vi "STC_Starrag_main_V3.vi"() -> ()   [LabVIEW 2017]
uses:
  controls/FPGA State.ctl
  controls/UI Data2.ctl
  controls/Chatter data.ctl
  Globals/Global - All UI Loop Stop.vi
  Globals/Global - UI Stream and Variable Connections.vi
  Globals/Global - Configuration Options.vi
  UI Error Handlers/support/User Event - Stop/User Event - Stop.lvlib
  UI Error Handlers/support/Message Queue/Message Queue.lvlib
panel:
  out "Raw Waveform":waveform(dbl)[](graph)
  in  "Settings Tab":T1(tab)=enum."Data Monitoring"
  in  "OK Button":bool
  in  "Tool Data File":path=path "K:/Core Research/Project Folders/AI Projects/AI3190 Digital Shop Floor Rollout/5 Software Files/Catapult/tool_path.txt"
  in  "Run Control":bool
  in  "Stop Control":bool
  in  "Max Acceleration Threshold (g)":sgl=0.03
  in  "In-cut Power Threshold":dbl=1.0
  in  "Controller Address":string="143.167.158.195"
  in  "Connect to Controller":bool
  out "Connected?":bool
  out "System Status":string
  in  "Save?":bool
  in  "Switch to Safe State":bool
  out "Current FPGA State":T2
  out "Tool Data":string="\n"
  in  "ODBC data source name":string="amrc_monitoring"
  in  "MT Connect Agent":string="http://amrcmtconnect.shef.ac.uk:5000/"
  in  "milliseconds to wait":u32=100
  in  "Machine":string="STC1250"
  out "Loop execution":u32
  out "output cluster":cluster{"G1 ":bool}
  out "tag acc":string
  out "tag spike":string
  out "Chatter?":bool
  out "Feed":dbl
  out "ACC  (grms)":T3(graph)
  out "Block of code being executed":string
  out "Program Name":string
  out "RPM":dbl
  out "STC Starrag":bool
  out "Force (grms)":T4(graph)
  out "Tool id":string
  out "Spindle Load":dbl[](graph)
  out "CPU Usage (%)":dbl[][](graph)
  out "Free Physical Memory or Largest Contiguous Memory (bytes)":dbl(graph)
  out "DMA FIFO Overflow?":bool
  in  "Exit":bool
  # "Acceleration Waveform for 0.5s"
  # "Connection Settings"
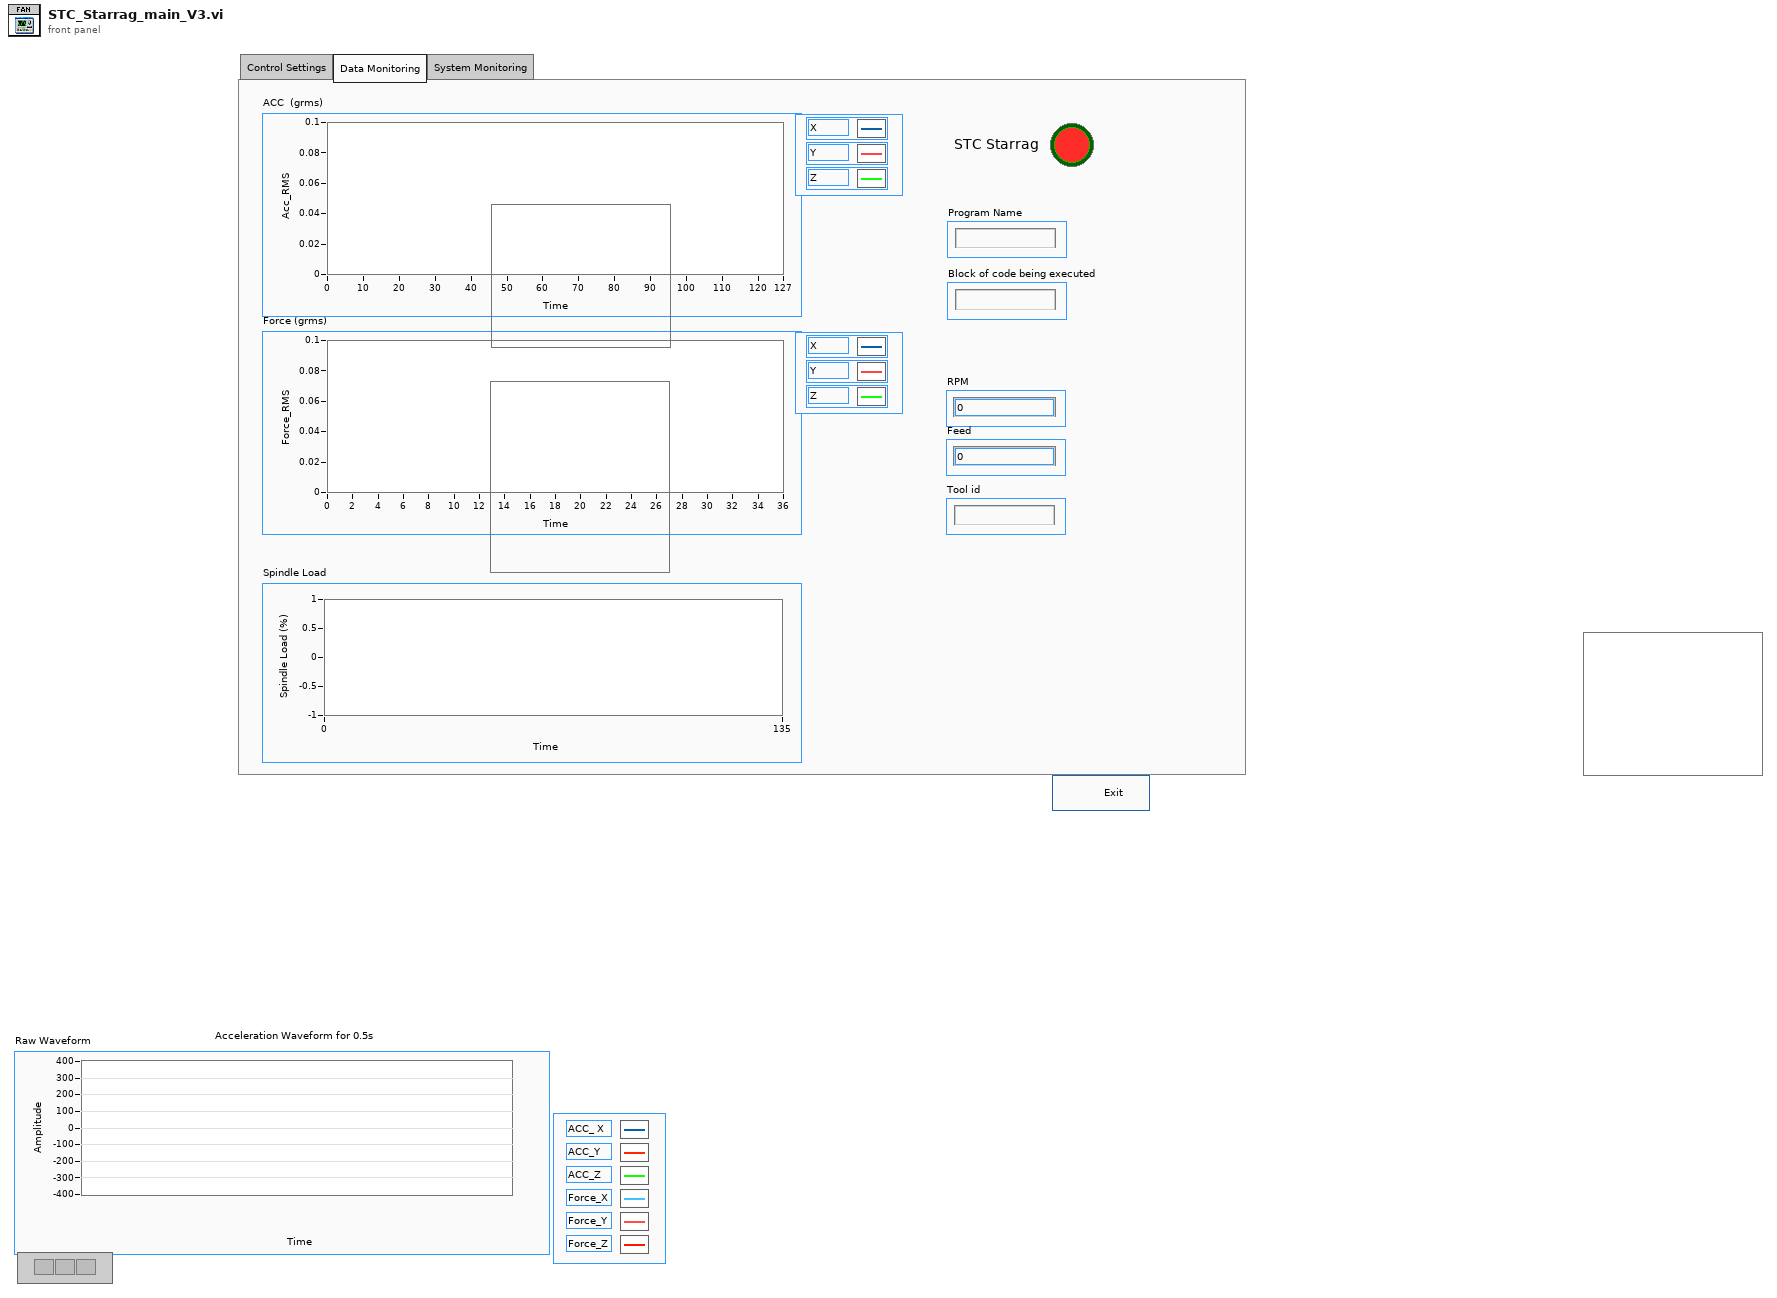
[diagram p1: front panel]
types:
  T1 = enum32{"Control Settings", "Data Monitoring", "System Monitoring"}
  T2 = typedef "FPGA State.ctl" = enum16{"Safe State", "Control (PID)"}
  T3 = cluster{"Array of Double[0]":dbl, "Array of Double[1]":dbl, "Array of Double[2]":dbl}
  T4 = cluster{"[0]":dbl, "[1]":dbl, "[2]":dbl, "[3]":dbl, "[4]":dbl, "[5]":dbl, "[6]":dbl, "[7]":dbl}
  T5 = typedef "UI Data2.ctl" = cluster{"Switch to Safe State Ref":refnum<vi>, "Run Control Ref":refnum<vi>, "Stop Control Ref":refnum<vi>, "Update Control Configurations Ref":refnum<vi>, "Chatter Data Ref":refnum<vi>, "Max Acceleration Threshold Ref":refnum<vi>}
  T6 = typedef "Message Queue.lvlib/All Message Queues.ctl" = cluster{"UI":refnum<queue>}
  T7 = enum8{"Enabled", "Disabled", "Disabled and Grayed Out"}
  T8 = cluster{"Message":string, "Message Data":variant}
  T9 = typedef "Chatter data.ctl" = cluster{"Tool data":cluster{"Number of teeth":sgl}, "Cutting data":cluster{"rpm":sgl}, "Limits":cluster{"Magnitude threshold":sgl, "Tolerance":sgl}, "G1 status":cluster{"G1 ":bool}}
  T10 = cluster{"FPGA State":T2, "Max Acceleration Threshold":sgl, "Chatter Data":T9}
  T11 = cluster{"seconds since 1Jan1904":timestamp, "number":dbl[][], "Machine Data":cluster{"Zload":string, "Yload":string, "Xload":string, "path_position":string, "Fovr":string, "SspeedOvr":string, "Program Name":string, "Program status":string, "Block of code being executed":string, "Line of code":string, "Machine availability":string, "Emergency status":string, "Controller mode":string, "Tool_id":string}}
  T12 = cluster{"seconds since 1Jan1904":timestamp, "number":dbl[][], "Machine Data":cluster{"Zload":string, "Yload":string, "Xload":string, "path_position":string, "Fovr":string, "SspeedOvr":string, "Program Name":string, "Program status":string, "Block of code being executed":string, "Line of code":string, "Machine availability":string, "Emergency status":string, "Controller mode":string, "Tool id":string}}
  T13 = cluster{"Actual PID Loop Period":refnum<k21>, "DMA FIFO Overflow?":refnum<k21>, "CPU Usage":refnum<k21>, "Free or Contiguous Memory":refnum<k21>, "Current FPGA State":refnum<k21>, "Acceleration (grms)":refnum<k21>, "Acceleration Waveform":refnum<k21>, "Chatter":refnum<k21>, "tag acc":refnum<k21>, "tag video":refnum<k21>, "Image Waveform":refnum<k21>}
  T14 = cluster{"Zload":string, "Yload":string, "Xload":string, "path_position":string, "Fovr":string, "SspeedOvr":string, "Program Name":string, "Program status":string, "Block of code being executed":string, "Line of code":string, "Machine availability":string, "Emergency status":string, "Controller mode":string, "Tool_id":string}
  T15 = cluster{"Zload":string, "Yload":string, "Xload":string, "path_position":string, "Fovr":string, "SspeedOvr":string, "Program Name":string, "Program status":string, "Block of code being executed":string, "Line of code":string, "Machine availability":string, "Emergency status":string, "Controller mode":string, "Tool id":string}
  T16 = cluster{"Magnitude threshold":sgl, "Tolerance":sgl}
  T17 = typedef "FPGA state.ctl" = enum16{"Safe State", "Control (PID)"}
  T18 = typedef "CPU Loads.ctl" = cluster{"Total (%)":dbl, "Time Critical (%)":dbl, "Timed Structures (%)":dbl, "High (%)":dbl, "Above Normal (%)":dbl, "Normal (%)":dbl, "Background (%)":dbl, "Idle (%)":dbl, "ISR (%)":dbl}[]
  T19 = cluster{"seconds since 1Jan1904":timestamp, "appended array":dbl[][], "Machine Data":cluster{"Zload":string, "Yload":string, "Xload":string, "path_position":string, "Fovr":string, "SspeedOvr":string, "Program Name":string, "Program status":string, "Block of code being executed":string, "Line of code":string, "Machine availability":string, "Emergency status":string, "Controller mode":string, "Tool_id":string}}
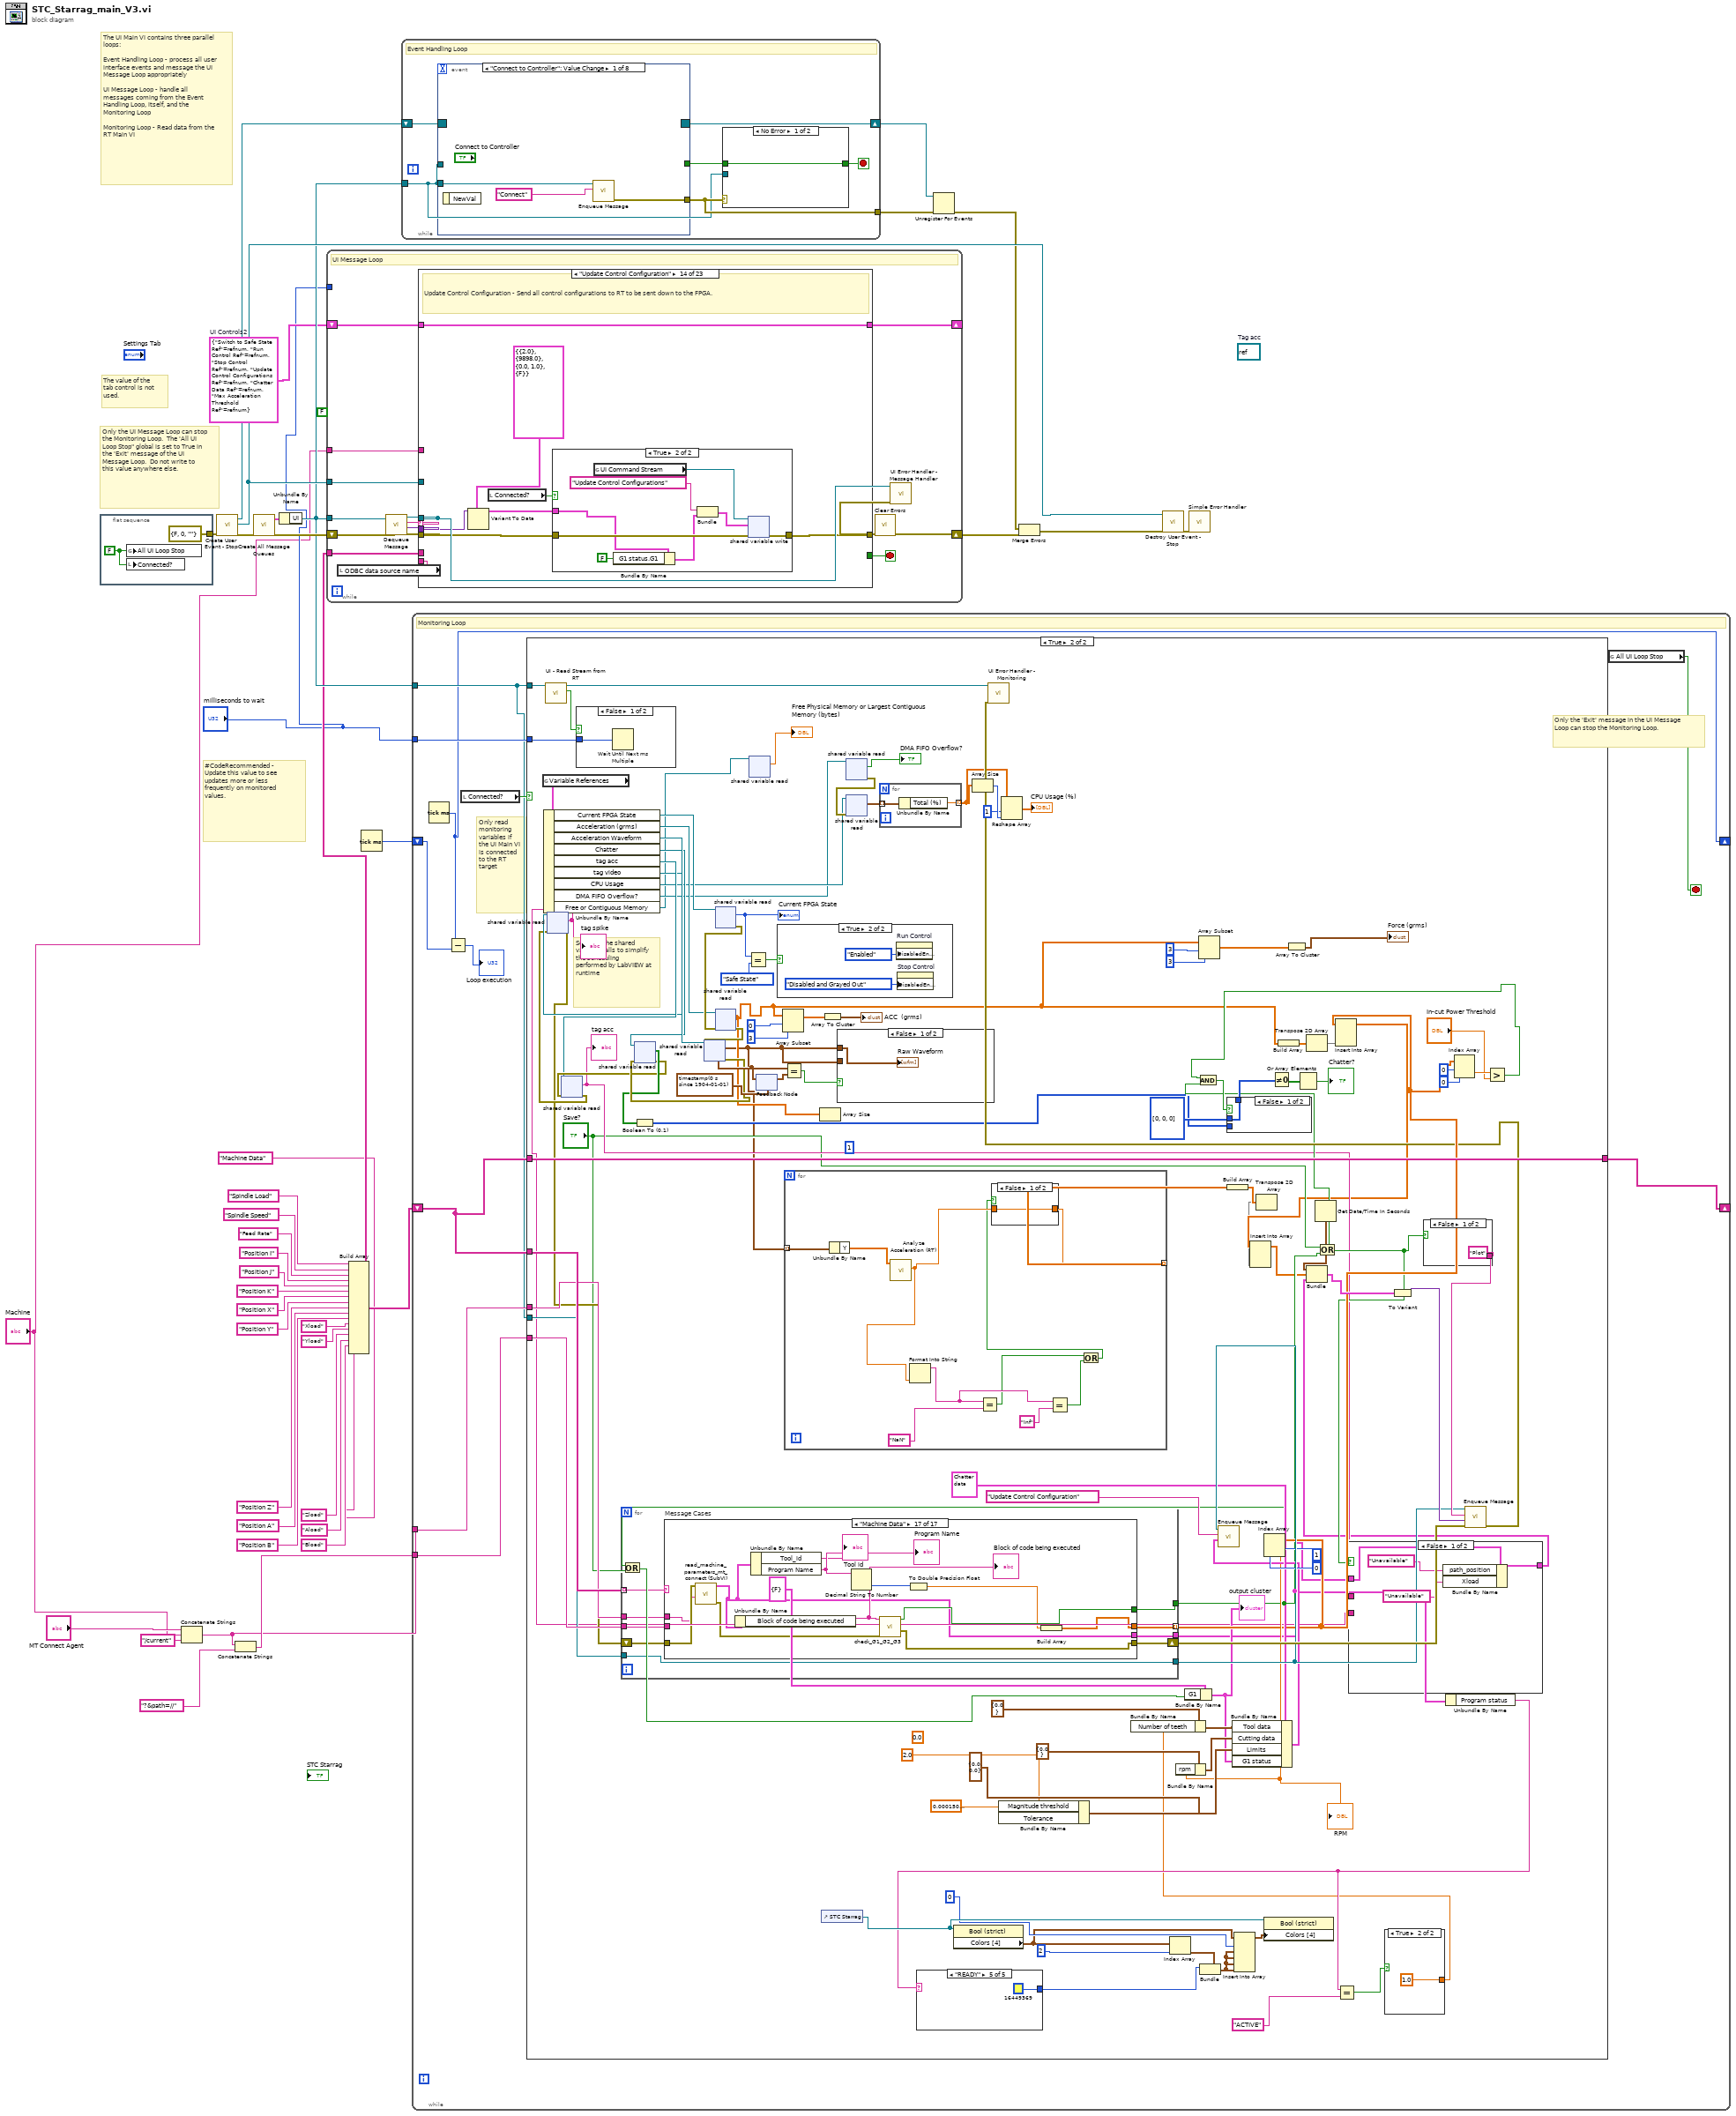
[diagram p0: block diagram]
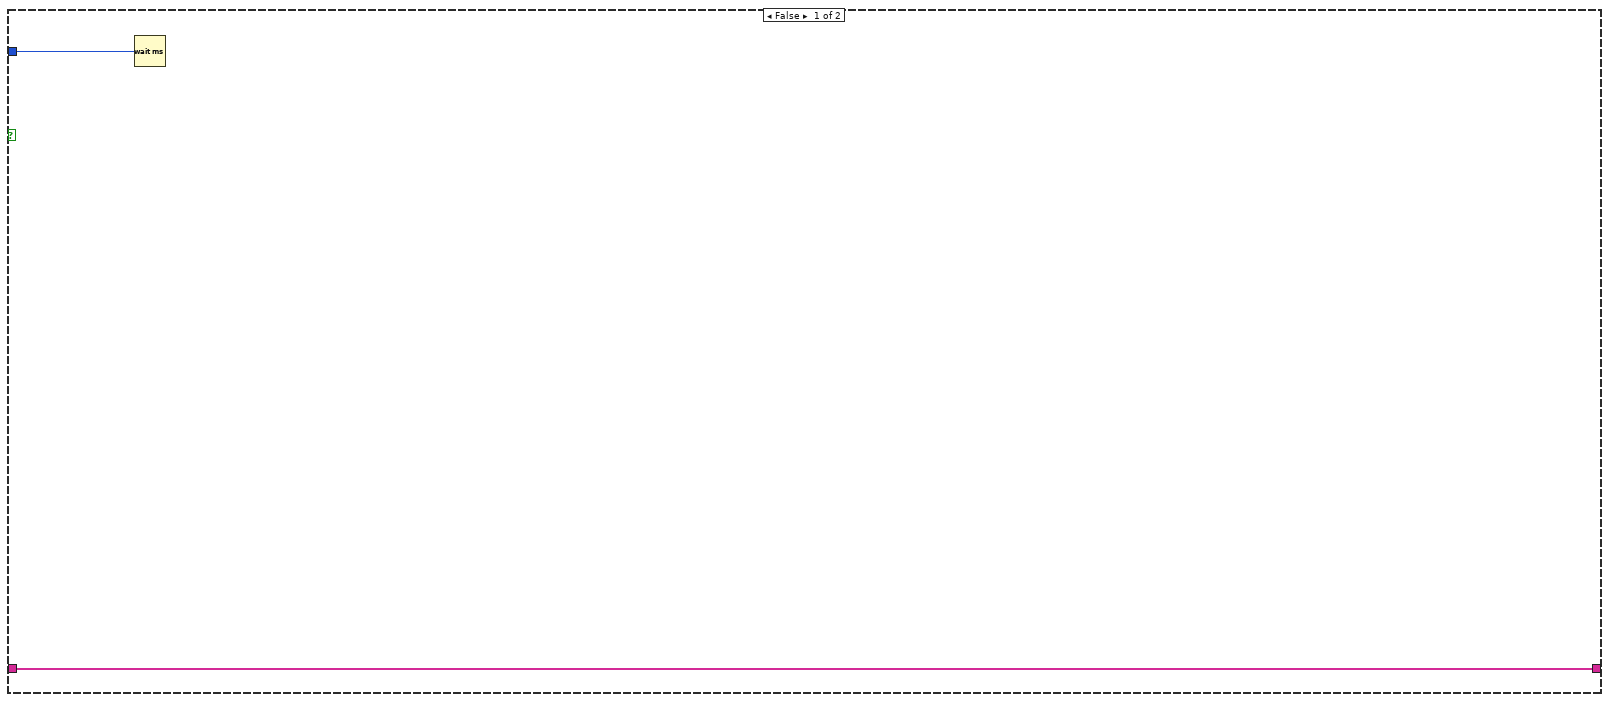
[diagram p2: hidden frame]
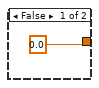
[diagram p3: hidden frame]
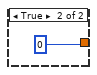
[diagram p4: hidden frame]
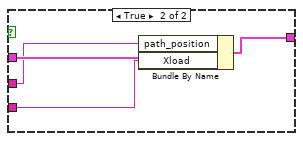
[diagram p5: hidden frame]
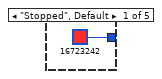
[diagram p6: hidden frame]
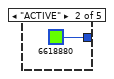
[diagram p7: hidden frame]
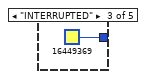
[diagram p8: hidden frame]
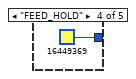
[diagram p9: hidden frame]
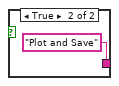
[diagram p11: hidden frame]
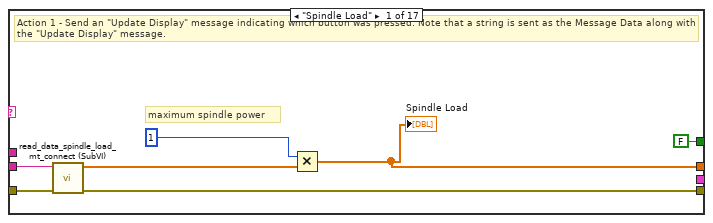
[diagram p12: hidden frame]
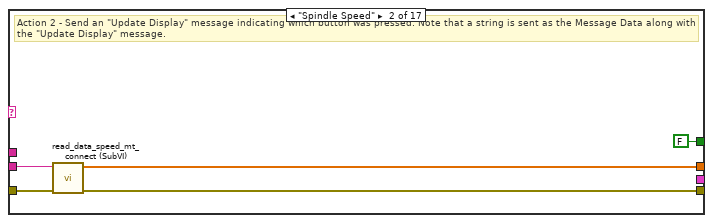
[diagram p13: hidden frame]
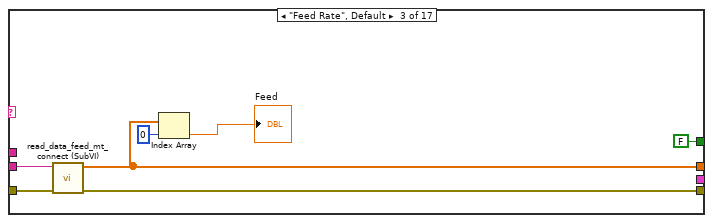
[diagram p14: hidden frame]
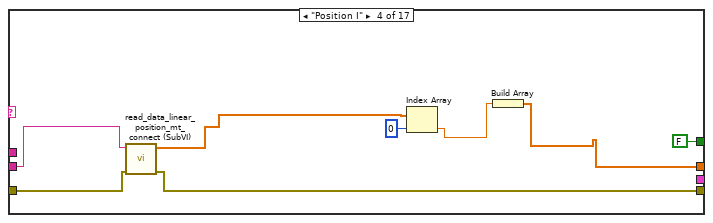
[diagram p15: hidden frame]
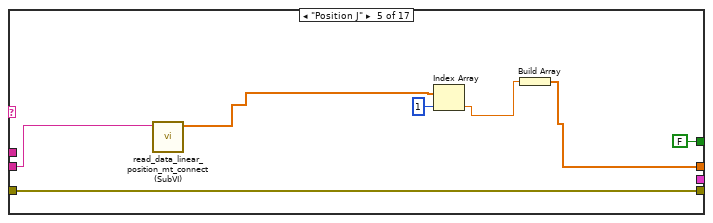
[diagram p16: hidden frame]
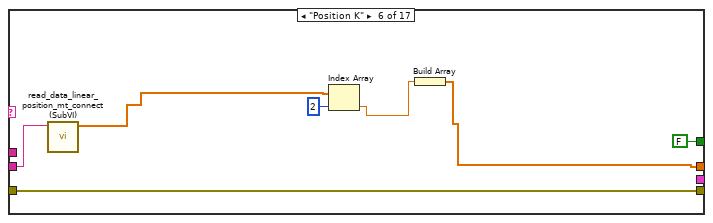
[diagram p17: hidden frame]
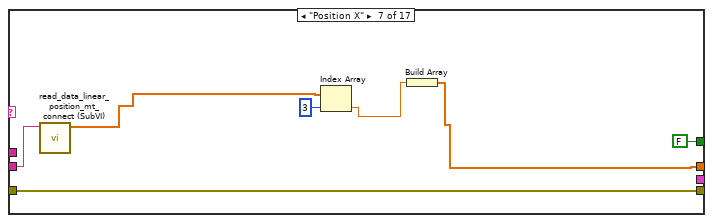
[diagram p18: hidden frame]
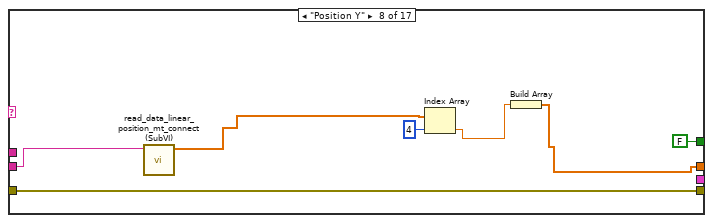
[diagram p19: hidden frame]
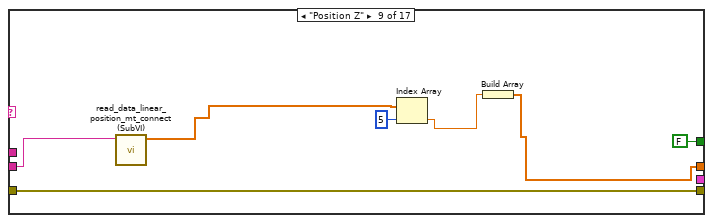
[diagram p20: hidden frame]
diagram:
  (unwired) refnum<k21> refnum  # Tag acc
  (unwired) FALSE ("Record  SS 661")
  w27 = T5 {"Switch to Safe State Ref"=refnum, "Run Control Ref"=refnum, "Stop Control Ref"=refnum, "Update Control Configurations Ref"=refnum, "Chatter Data Ref"=refnum, "Max Acceleration Threshold Ref"=refnum}  # UI Controls2
  # "#CodeRecommended - Update this value to see updates more or less frequently on monitored values."
  # "The UI Main VI contains three parallel loops:\n\nEvent Handling Loop - process all user interface events and message the UI Message Loop appropriately\n\nUI Message Loop - handle all messages coming from the Event Handling Loop, itself, and the Monitoring Loop\n\nMonitoring Loop - Read data from the RT Main VI"
  # "The value of the tab control is not used."
  # "Only the UI Message Loop can stop the Monitoring Loop.  The 'All UI Loop Stop\" global is set to True in the 'Exit' message of the UI Message Loop.  Do not write to this value anywhere else."
  n1 = flat-sequence {
    tunnel: [errorcluster {"status"=FALSE, "code"=0, "source"=""} ("error in (no error)")] -> w28
    frame #0 {
      w41 = FALSE
      n2 = global write "Global - All UI Loop Stop.vi" "All UI Loop Stop"(w41) -> ()
      n3 = local write "Connected?"(w41) -> ()
    }
  }
  n4 = Concatenate Strings("MT Connect Agent", "Machine", "/current" ("string")) -> (w18:string)
  n5 = call "Create User Event - Stop.vi"("error in (no error)"=w28) -> ("error out"=w35:errorcluster, "User Event - Stop"=w36:refnum<user-event>, "Stop Event Registration Refnum"=w37:refnum<event-registration>)  [unwired: 8 in]
  n6 = Concatenate Strings(w18, "?&path=//" ("string")) -> (w22:string)
  n7 = call "Create All Message Queues.vi"("error in (no error)"=w35) -> ("error out"=w33:errorcluster, "Message Queues out"=w34:T6)  [unwired: 9 in]
  n8 = Unbundle By Name(w34) -> ("UI"=w29:refnum<queue>)
  n9 = Build Array("Spindle Load" ("Message"), "Spindle Speed" ("Message"), "Feed Rate" ("element"), "Position I" ("element"), "Position J" ("element"), "Position K" ("element"), "Position X" ("element"), "Position Y" ("element"), "Position Z" ("element"), "Position A" ("element"), "Position B" ("element"), "Xload" ("element"), "Yload" ("element"), "Zload" ("element"), "Aload" ("element"), "Bload" ("element"), "Machine Data" ("element")) -> (w21:string[])
  n10 = while {
    tunnel: w29 -> [w51]
    tunnel: w36 -> [w56]
    shift-right: [w46] -> w40
    shift-left: w33 -> [w55]
    shift-right: [w49] -> _
    shift-left: w27 -> [w50]
    tunnel: w21 -> [w45]
    tunnel: "Machine" -> [w44]
    tunnel: "milliseconds to wait" -> [_]
    stop <- w57 stop-if-true
    # "UI Message Loop"
    n11 = local read "ODBC data source name"() -> (w43:string)
    n12 = call "Dequeue Message.vi"("error in (no error)"=w55, "Message Queue"=w51) -> ("error out"=w54:errorcluster, "Message Data"=w52:variant, "Message"=w53:string, "dup Message Queue"=w48:refnum<queue>)  [unwired: 6 in]
    n13 = case "Message Cases" shown="\"Update Control Configuration\"" w53 {
      selector: w53 -> [_ _ _ _ _ _ _ _ _ _ _ _ w192 _ w228 _ w263 _ _ _ _ _ w362]
      tunnel: w48 -> [w59 w65 _ _ w98 _ w116 w124 _ w149 _ _ w193 _ _ _ w267 _ w310 _ _ w336 _]
      tunnel: w54 -> [w61 w72 w85 w91 w103 w114 w118 w122 w138 w158 w174 w189 w195 w213 w229 w247 w277 w298 w315 w320 w332 w337 _]
      tunnel: [w60 w66 w85 w91 w97 w114 w117 w127 w137 w151 w163 w177 w194 w215 w230 w246 w278 w296 w316 w319 w331 w340 w360] -> w47
      tunnel: [_ _ _ _ _ _ _ _ _ _ _ _ _ _ _ _ _ _ TRUE _ _ _ _] -> w57
      tunnel: w52 -> [_ _ _ _ _ _ _ _ _ w156 w173 w188 _ w212 w227 w245 w275 w295 _ _ w329 _ _]
      tunnel: w56 -> [_ _ _ _ _ _ _ _ _ _ _ _ _ _ _ _ _ _ w314 _ _ _ _]
      tunnel: w50 -> [w62 w71 w84 w93 w102 w113 w120 w128 w139 w154 w175 w190 w196 w216 w231 w244 w279 w297 w312 w318 w330 w339 w358]
      tunnel: [w62 w70 w84 w93 w102 w113 w120 w128 w139 w154 w175 w190 w196 w216 w231 w244 w279 w297 w312 w318 w330 w339 w358] -> w49
      tunnel: w45 -> [_ _ _ _ _ _ _ _ _ _ _ _ _ _ _ _ _ _ _ _ _ _ _]
      tunnel: w43 -> [_ _ _ _ _ _ _ _ _ _ w162 w176 _ _ _ _ _ _ _ _ _ _ _]
      tunnel: w44 -> [_ _ _ _ _ _ _ _ _ _ w167 w182 _ _ _ _ _ _ _ _ _ _ _]
      frame "Initialize" {
        # "Initialize - Send 'Initialize UI Refs' message to get the UI references bundled and initialized appropriately."
        n14 = call "Enqueue Message.vi"("error in (no error)"=w61, "Message"="Initialize UI Refs", "Message Queue"=w59) -> ("error out"=w60:errorcluster)  [unwired: 7 in, 1 out]
      }
      frame "Initialize UI Refs" {
        # "Send a message to disable them all, since there is no connection at the start."
        # "Initialize UI Refs - Bundle up a cluster of references of all UI elements that are programmatically manipulated."
        n15 = control-ref of="Max Acceleration Threshold (g)"() -> (w63:refnum<vi>)
        n16 = control-ref of="Switch to Safe State"() -> (w69:refnum<vi>)
        n17 = control-ref of="Run Control"() -> (w68:refnum<vi>)
        n18 = control-ref of="Stop Control"() -> (w67:refnum<vi>)
        n19 = call "Enqueue Message.vi"("error in (no error)"=w72, "Message"="Disable Controls", "Message Queue"=w65) -> ("error out"=w66:errorcluster)  [unwired: 7 in, 1 out]
        n20 = Bundle By Name(cluster=w71, "Switch to Safe State Ref"=w69, "Run Control Ref"=w68, "Stop Control Ref"=w67, "Max Acceleration Threshold Ref"=w63) -> (w70:T5)
      }
      frame "Disable Controls" {
        w75 = 0
        # "With the control options disabled, the only thing the user can do is Connect. Make sure the IP address string and connect button are enabled."
        # "Disable All Controls - Set all controls in the UI Refs cluster to \"Disabled and Grayed Out\"."
        n21 = Unbundle(w84) -> ("Switch to Safe State Ref"=w83:refnum<vi>, "Run Control Ref"=w82:refnum<vi>, "Stop Control Ref"=w81:refnum<vi>, "Update Control Configurations Ref"=w80:refnum<vi>, "Chatter Data Ref"=w79:refnum<vi>, "Max Acceleration Threshold Ref"=w78:refnum<vi>)
        n22 = Build Array(w83, w82, w81, w80, w79, w78) -> (w77:refnum<vi>[])
        n23 = property on="ODBC data source name" class="Str"("DisabledEnum"=T7."Enabled" ("Disabled")) -> ()  [unwired: 2 in, 2 out]
        n24 = property on="In-cut Power Threshold" class="DigNum (strict)"("DisabledEnum"=T7."Disabled and Grayed Out" ("Disabled")) -> ()  [unwired: 2 in, 2 out]
        n25 = call "Set Enable State on Multiple Controls.vi"("Enable?"=FALSE, "Controls"=w77) -> ()  [unwired: 10 in]
        n26 = property on="Controller Address" class="Str"("DisabledEnum"=w75) -> ()  [unwired: 2 in, 2 out]
        n27 = property on="Connect to Controller" class="Bool"("DisabledEnum"=w75) -> ()  [unwired: 2 in, 2 out]
      }
      frame "Enable Configuration Controls" {
        w94 = 2
        # "Once connected, the user shouldn't be able to change the connection settings unless he gets disconnected."
        # "Enable Configuration Controls - After successful connection, ensure appropriate controls are enabled."
        n28 = Unbundle By Name(w93) -> ("Update Control Configurations Ref"=w92:refnum<vi>, "Max Acceleration Threshold Ref"=w90:refnum<vi>, "Chatter Data Ref"=w89:refnum<vi>, "Switch to Safe State Ref"=w88:refnum<vi>)
        n29 = property on="In-cut Power Threshold" class="DigNum (strict)"("DisabledEnum"=T7."Enabled" ("Disabled")) -> ()  [unwired: 2 in, 2 out]
        n30 = property on="ODBC data source name" class="Str"("DisabledEnum"=T7."Disabled and Grayed Out" ("Disabled")) -> ()  [unwired: 2 in, 2 out]
        n31 = Build Array(w92, w90, w89, w88) -> (w96:refnum<vi>[])
        n32 = call "Set Enable State on Multiple Controls.vi"("Enable?"=TRUE, "Controls"=w96) -> ()  [unwired: 10 in]
        n33 = property on="Controller Address" class="Str"("DisabledEnum"=w94) -> ()  [unwired: 2 in, 2 out]
        n34 = property on="Connect to Controller" class="Bool"("DisabledEnum"=w94) -> ()  [unwired: 2 in, 2 out]
      }
      frame "Connect" {
        # "Connect - Attempt to connect to both streams, and the variables, on the RT target."
        n35 = call "UI - Initiate Connection.vi"("error in (no error)"=w103, "Controller Address"="Controller Address", "Message Queue"=w98) -> ("error out"=w100:errorcluster, "Connected?"=w99:bool)  [unwired: 7 in]
        "Connected?" <- w99
        n36 = case shown="True" w99 {
          tunnel: w100 -> [w104 w108]
          tunnel: w98 -> [_ w107]
          tunnel: [w104 w106] -> w97
          frame False {
          }
          frame True {
            n37 = call "Enqueue Message.vi"("error in (no error)"=w108, "Message"="Enable Configuration Controls", "Message Queue"=w107) -> ("error out"=w106:errorcluster)  [unwired: 7 in, 1 out]
          }
        }
      }
      frame "Close Connections" {
        # "Close Connections - Close the connections shared with the Monitoring Loop."
        n38 = global read "Global - UI Stream and Variable Connections.vi" "UI Command Stream"() -> (w112:refnum<k21>)
        n39 = global read "Global - UI Stream and Variable Connections.vi" "RT Message Stream"() -> (w111:refnum<k21>)
        n40 = global read "Global - UI Stream and Variable Connections.vi" "Variable References"() -> (w109:T13)
        n41 = local write "Connected?"(FALSE ("Connected?")) -> ()
        n42 = Destroy Stream Endpoint(11:w112) -> ()  [unwired: 1 in, 1 out]
        n43 = Destroy Stream Endpoint(11:w111) -> ()  [unwired: 1 in, 1 out]
        n44 = call "Close Variable Connections.vi"("Variable References 2"=w109) -> ()  [unwired: 11 in]
      }
      frame "Disconnect UI" {
        # "Disable Controls"
        # "Disconnect UI - Something has gone wrong with the connection. Reinitialize the UI to its disconnected state."
        n45 = local write "Connected?"(FALSE ("Connected?")) -> ()
        n46 = call "Enqueue Message.vi"("error in (no error)"=w118, "Message"="Reconnect", "Message Queue"=w116) -> ("error out"=w117:errorcluster)  [unwired: 7 in, 1 out]
      }
      frame "Reconnect" {
        # "Disconnect UI - Something has gone wrong with the connection. Reinitialize the UI to its disconnected state."
        n47 = Flush Queue(queue=w124, error in (no error)=w122) -> (queue out=w123:refnum<queue>, error out=w121:errorcluster)  [unwired: 1 out]
        n48 = flat-sequence {
          tunnel: w123 -> [w130]
          tunnel: w121 -> [w131]
          tunnel: [w131] -> w126
          tunnel: [w130] -> w125
          tunnel: w126 -> [w134]
          tunnel: w125 -> [w132]
          tunnel: [w133] -> w127
          frame #0 {
            n49 = Wait Until Next ms Multiple(millisecond multiple=u32 10000) -> ()  [unwired: 1 out]
          }
          frame #1 {
            n50 = call "Enqueue Message.vi"("error in (no error)"=w134, "Message"="Connect", "Message Queue"=w132) -> ("error out"=w133:errorcluster)  [unwired: 7 in, 1 out]
          }
        }
      }
      frame "Get Settings from FPGA" {
        # "Get Settings from FPGA - Send a command to the RT to retrieve all current FPGA Main VI parameter values and send them back to the UI."
        n51 = local read "Connected?"() -> (w136:bool)
        n52 = case shown="True" w136 {
          tunnel: w138 -> [w140 w144]
          tunnel: [w140 w143] -> w137
          frame False {
            # "Don't bother trying to send a message to the RT system if UI Main VI isn't even connected"
          }
          frame True {
            n53 = global read "Global - UI Stream and Variable Connections.vi" "UI Command Stream"() -> (w141:refnum<k21>)
            n54 = shared-variable-write(w141, w144, T8 {"Message"="Send FPGA Configuration to UI", "Message Data"=variant} ("data in")) -> (w143:errorcluster)  [unwired: 1 in, 2 out]
          }
        }
      }
      frame "Initial UI Values" {
        # "Set values of all manual and setpoint controls via reference."
        # "Initial UI Values - These are the current values of the FPGA Main VI's R/W controls. They are used to initialize the panel of UI Main VI upon successful connection to the RT target."
        n55 = Variant To Data(error in=w158, type=T10 {"FPGA State"=enum."Safe State", "Max Acceleration Threshold"=0.0, "Chatter Data"={"Tool data"={"Number of teeth"=2.0}, "Cutting data"={"rpm"=9898.0}, "Limits"={"Magnitude threshold"=0.0, "Tolerance"=1.0}, "G1 status"={"G1 "=FALSE}}}, Variant=w156) -> (data=w155:T10, error out=w157:errorcluster)
        n56 = Unbundle By Name(w154) -> ("Max Acceleration Threshold Ref"=w146:refnum<vi>)
        n57 = Unbundle By Name(w155) -> ("Max Acceleration Threshold"=w148:sgl, "FPGA State"=w147:T2)  [unwired: 1 out]
        n58 = Build Array(w146, w146) -> (w153:refnum<vi>[])
        n59 = Build Array(w148) -> (w152:sgl[])
        n60 = for {
          tunnel: w153 -> [w160] mode=indexing
          tunnel: w152 -> [w159] mode=indexing
          n61 = property class="DigNum (strict)"(reference=w160, "Value"=w159) -> ()  [unwired: 1 in, 2 out]
        }
        n62 = local write "Current FPGA State"(w147) -> ()
        n63 = call "Enqueue Message.vi"("error in (no error)"=w157, "Message Data"=w147, "Message"="Update Display Mode", "Message Queue"=w149) -> ("error out"=w151:errorcluster)  [unwired: 6 in, 1 out]
      }
      frame "Plot and Save" {
        n64 = Variant To Data(error in=w174, type=T11 {"seconds since 1Jan1904"=timestamp(0 s since 1904-01-01), "number"=[], "Machine Data"={"Zload"="", "Yload"="", "Xload"="", "path_position"="", "Fovr"="", "SspeedOvr"="", "Program Name"="", "Program status"="", "Block of code being executed"="", "Line of code"="", "Machine availability"="", "Emergency status"="", "Controller mode"="", "Tool_id"=""}} ("output cluster"), Variant=w173) -> (data=w172:T11, error out=w164:errorcluster)
        n65 = Unbundle(w172) -> ("seconds since 1Jan1904"=w165:timestamp, "number"=w170:dbl[][], "Machine Data"=w168:T14)
        n66 = Index Array(array=w170, index (col)=0 ("disabled index (col)")) -> (element=w161:dbl[])  [unwired: 1 in]
        n67 = call "database_connection_write_DMMS_2.vi"("ODBC data source name"=w162, "error in (no error)"=w164, "G1?"=u32 1, "current time"=w165, "data 2"=w161, "Machine Data"=w168, "Machine type"=w167) -> ("error out"=w163:errorcluster)  [unwired: 4 in]
      }
      frame "Plot" {
        (unwired) u32 0 ("G1?")
        n68 = Variant To Data(error in=w189, type=T12 {"seconds since 1Jan1904"=timestamp(0 s since 1904-01-01), "number"=[], "Machine Data"={"Zload"="", "Yload"="", "Xload"="", "path_position"="", "Fovr"="", "SspeedOvr"="", "Program Name"="", "Program status"="", "Block of code being executed"="", "Line of code"="", "Machine availability"="", "Emergency status"="", "Controller mode"="", "Tool id"=""}} ("output cluster"), Variant=w188) -> (data=w186:T12, error out=w178:errorcluster)
        n69 = Unbundle(w186) -> ("seconds since 1Jan1904"=w180:timestamp, "number"=w184:dbl[][], "Machine Data"=w181:T15)
        n70 = Index Array(array=w184, index (col)=0 ("disabled index (col)")) -> (element=w183:dbl[])  [unwired: 1 in]
        n71 = call "database_connection_write_DMMS_2.vi"("ODBC data source name"=w176, "error in (no error)"=w178, "G1?"=u32 0, "current time"=w180, "data 2"=w183, "Machine Data"=w181, "Machine type"=w182) -> ("error out"=w177:errorcluster)  [unwired: 4 in]
      }
      frame "Run Control", "Run Safe State", "Stop Control" {
        # "Run/Stop buttons - Send a command to switch the FPGA into the appropriate state. Send a message to update this UI to reflect the new state."
        n72 = local read "Connected?"() -> (w191:bool)
        n73 = case shown="False" w191 {
          tunnel: w195 -> [w197 w207]
          tunnel: [w197 w203] -> w194
          tunnel: w193 -> [_ w202]
          tunnel: w192 -> [_ w201]
          frame False {
            # "Don't bother trying to send a message to the RT system if UI Main VI isn't even connected"
          }
          frame True {
            # "Run Control switch into Run Control state. Anything else switches to Safe State."
            n74 = case shown="\"Run Control\"" w201 {
              tunnel: [FPGA_State."Safe State" ("FPGA State") FPGA_State."Control (PID)" ("FPGA State")] -> w198
              frame "Safe State", "Stop Control", Default {
              }
              frame "Run Control" {
              }
            }
            n75 = global read "Global - UI Stream and Variable Connections.vi" "UI Command Stream"() -> (w199:refnum<k21>)
            n76 = Bundle("Update FPGA State", "FPGA State"=w198) -> (w204:cluster{string, "FPGA State":T2})  [unwired: 1 in]
            n77 = shared-variable-write(w199, w207, w204) -> (w206:errorcluster)  [unwired: 1 in, 2 out]
            n78 = call "Enqueue Message.vi"("error in (no error)"=w206, "Message Data"=w198, "Message"="Update Display Mode", "Message Queue"=w202) -> ("error out"=w203:errorcluster)  [unwired: 6 in, 1 out]
          }
        }
      }
      frame "Update Control Configuration" {
        # "Update Control Configuration - Send all control configurations to RT to be sent down to the FPGA."
        n79 = Variant To Data(type=T9 {"Tool data"={"Number of teeth"=2.0}, "Cutting data"={"rpm"=9898.0}, "Limits"={"Magnitude threshold"=0.0, "Tolerance"=1.0}, "G1 status"={"G1 "=FALSE}} ("Chatter Data"), Variant=w212) -> (data=w211:T9)  [unwired: 1 in, 1 out]
        n80 = local read "Connected?"() -> (w214:bool)
        n81 = case shown="True" w214 {
          tunnel: w213 -> [w217 w225]
          tunnel: [w217 w224] -> w215
          tunnel: w211 -> [_ w220]
          frame False {
            # "Don't bother trying to send a message to the RT system if UI Main VI isn't even connected"
          }
          frame True {
            n82 = global read "Global - UI Stream and Variable Connections.vi" "UI Command Stream"() -> (w221:refnum<k21>)
            n83 = Bundle By Name(cluster=w220, "G1 status.G1"=FALSE) -> (w218:T9)
            n84 = Bundle("Update Control Configurations", "Chatter Data"=w218) -> (w222:cluster{string, "Chatter Data":T9})  [unwired: 1 in]
            n85 = shared-variable-write(w221, w225, w222) -> (w224:errorcluster)  [unwired: 1 in, 2 out]
          }
        }
      }
      frame "Update Max Acceleration Threshold", "Update Max Fan Speed Threshold", "Update Setpoints" {
        # "Update Manual Values/Setpoints - Send all manual values/setpoints to RT to be sent down to the FPGA."
        n86 = local read "Connected?"() -> (w226:bool)
        n87 = case shown="True" w226 {
          tunnel: [w232 w238] -> w230
          tunnel: w229 -> [w232 w236]
          tunnel: w228 -> [_ w235]
          tunnel: w227 -> [_ w234]
          frame False {
            # "Don't bother trying to send a message to the RT system if UI Main VI isn't even connected"
          }
          frame True {
            n88 = global read "Global - UI Stream and Variable Connections.vi" "UI Command Stream"() -> (w233:refnum<k21>)
            n89 = Bundle(w235, "Message Data"=w234) -> (w237:cluster{string, "Message Data":variant})  [unwired: 1 in]
            n90 = shared-variable-write(w233, w236, w237) -> (w238:errorcluster)  [unwired: 1 in, 2 out]
          }
        }
      }
      frame "Update Display Mode" {
        # "Update Display Mode - Enable/Disable Controls appropriately for the new display mode."
        n91 = Variant To Data(error in=w247, type=FPGA_State."Safe State" ("FPGA State"), Variant=w245) -> (data=w243:T2, error out=w246:errorcluster)
        n92 = Unbundle By Name(w244) -> ("Switch to Safe State Ref"=w242:refnum<vi>, "Stop Control Ref"=w240:refnum<vi>, "Run Control Ref"=w239:refnum<vi>)
        n93 = case shown="\"Control (PID)\"" w243 {
          tunnel: w242 -> [w250 w256]
          tunnel: w239 -> [w248 w257]
          tunnel: w240 -> [w249 w255]
          frame "Control (PID)" {
            n94 = Build Array "Controls to Enable"(w250, w249) -> (w254:refnum<vi>[])
            n95 = Build Array "Controls to Disable"(w248) -> (w252:refnum<vi>[])
            n96 = call "Set Enable State on Multiple Controls.vi"("Enable?"=FALSE, "Controls"=w252) -> ()  [unwired: 10 in]
            n97 = call "Set Enable State on Multiple Controls.vi"("Enable?"=TRUE, "Controls"=w254) -> ()  [unwired: 10 in]
          }
          frame "Safe State", Default {
            # "This frame runs when FPGA is in Safe State. Only enable the run button."
            n98 = Build Array "Controls to Enable"(w257) -> (w261:refnum<vi>[])
            n99 = Build Array "Controls to Disable"(w256, w255) -> (w259:refnum<vi>[])
            n100 = call "Set Enable State on Multiple Controls.vi"("Enable?"=FALSE, "Controls"=w259) -> ()  [unwired: 10 in]
            n101 = call "Set Enable State on Multiple Controls.vi"("Enable?"=TRUE, "Controls"=w261) -> ()  [unwired: 10 in]
          }
        }
      }
      frame "Critical Error", "Log-Only Error", "Non-Critical Error", "RT Error" {
        # "Error - Display message in status indicator on panel.  If it's a critical error, shut down this VI with an 'Exit' message."
        n102 = case shown="Default" w263 {
          selector: w263 -> [_ w281]
          tunnel: ["UI Error" w281] -> w262
          frame Default {
          }
          frame "RT Error" {
          }
        }
        n103 = Variant To Data(error in=w277, type=errorcluster {"status"=FALSE, "code"=0, "source"=""} ("error constant"), Variant=w275) -> (data=w270:errorcluster, error out=w276:errorcluster)
        n104 = Unbundle By Name(w270) -> ("code"=w269:i32, "source"=w273:string)
        n105 = Format Date/Time String() -> (date/time string=w272:string)  [unwired: 3 in]
        n106 = Format Into String(format string="\n%s: %s %d - %s", w272, w262, w269, w273) -> (resulting string=w264:string)  [unwired: 2 in, 1 out]
        n107 = call "Enqueue Message.vi"("error in (no error)"=w276, "Message Data"=w264, "Message"="Update System Status", "Message Queue"=w267) -> ("error out"=w268:errorcluster, "dup Message Queue"=w266:refnum<queue>)  [unwired: 6 in]
        n108 = case shown="Default" w263 {
          tunnel: w268 -> [w282 w286]
          tunnel: w266 -> [_ w284]
          tunnel: [w282 w285] -> w278
          frame Default {
          }
          frame "Critical Error" {
            n109 = call "Enqueue Message.vi"("error in (no error)"=w286, "Message"="Exit", "Message Queue"=w284) -> ("error out"=w285:errorcluster)  [unwired: 7 in, 1 out]
          }
        }
      }
      frame "Update System Status" {
        # "#CodeRecommended - The code below ensures that the System Status string value does not become too large.  It uses the same maximum size as the RT error log to determine whether or not to remove the last half of the log string. Change this logic if you wish to maintain more/less of the information in the System Status string."
        # "Update System Status - Add a new string to the beginning of the System Status string on the UI."
        n110 = Variant To Data(error in=w298, type="", Variant=w295) -> (data=w292:string, error out=w296:errorcluster)
        n111 = local read "System Status"() -> (w290:string)
        n112 = global read "Global - Configuration Options.vi" "Error Log Max Size (bytes)"() -> (w288:i64)
        n113 = String Length(string=w290) -> (length=w291:i32)
        n114 = Greater?(x=w291, y=w288) -> (0:w289:bool)
        n115 = case shown="False" w289 {
          tunnel: w290 -> [w299 w303]
          tunnel: w288 -> [_ w302]
          tunnel: [w299 w304] -> w287
          frame False {
          }
          frame True {
            n116 = Divide(x=w302, y=i64 2) -> (x/y=w301:dbl)
            n117 = String Subset(string=w303, length (rest)=w301) -> (substring=w304:string)  [unwired: 1 in]
          }
        }
        n118 = Concatenate Strings(w292, w287) -> (→"System Status":string)
      }
      frame "Exit" {
        # "Close all connections"
        # "Stop Monitoring Loop"
        # "Stop Event Handling Loop"
        # "Release the UI Message queue reference"
        # "Stop UI Message Loop"
        # "Exit - Fire the User Event to stop the Event Handling Loop, and toggle the local variable to stop the Monitoring Loop.  This message alone causes all three loops to stop."
        n119 = local write "Connected?"(FALSE ("Connected?")) -> ()
        n120 = global write "Global - All UI Loop Stop.vi" "All UI Loop Stop"(TRUE ("Stop Monitoring Loop")) -> ()
        n121 = call "Fire User Event - Stop.vi"("User Event - Stop"=w314) -> ("error out"=w313:errorcluster)  [unwired: 10 in]
        n122 = Release Queue(queue=w310, error in (no error)=w315) -> (error out=w311:errorcluster)  [unwired: 1 in, 2 out]
        n123 = global read "Global - UI Stream and Variable Connections.vi" "UI Command Stream"() -> (w309:refnum<k21>)
        n124 = global read "Global - UI Stream and Variable Connections.vi" "RT Message Stream"() -> (w308:refnum<k21>)
        n125 = global read "Global - UI Stream and Variable Connections.vi" "Variable References"() -> (w305:T13)
        n126 = Destroy Stream Endpoint(11:w309) -> ()  [unwired: 1 in, 1 out]
        n127 = Destroy Stream Endpoint(11:w308) -> ()  [unwired: 1 in, 1 out]
        n128 = call "Close Variable Connections.vi"("Variable References 2"=w305) -> ()  [unwired: 11 in]
        n129 = Merge Errors(w313, w311) -> (w316:errorcluster)
      }
      frame "---Copy This Frame---" {
        # "Duplicate this frame when creating new messages.  Change this comment in the duplicated frame to describe this message."
        n130 = Merge Errors(w320) -> (w319:errorcluster)
      }
      frame "Update Tool Data" {
        # "Duplicate this frame when creating new messages.  Change this comment in the duplicated frame to describe this message."
        n131 = Variant To Data(type=path "" ("Tool Data File"), Variant=w329) -> (data=w321:path, error out=w323:errorcluster)  [unwired: 1 in]
        n132 = Build Path(name or relative path=w321) -> (appended path=w327:path)  [unwired: 1 in]
        n133 = Read from Text File(file (use dialog)=w327, error in=w323) -> (text=w324:string, error out=w326:errorcluster)  [unwired: 2 in, 2 out]
        n134 = Unbundle By Name(w326) -> ("status"=w325:bool)  [unwired: 1 out]
        n135 = case shown="False" w325 {
          tunnel: w324 -> [w333 _]
          tunnel: [w333 "Error"] -> w322
          frame False {
          }
          frame True {
          }
        }
        "Tool Data" <- w322
        n136 = Merge Errors(w332) -> (w331:errorcluster)
      }
      frame "Unsuccessful Connection" {
        # "Duplicate this frame when creating new messages.  Change this comment in the duplicated frame to describe this message."
        n137 = flat-sequence {
          tunnel: w339 -> [w342]
          tunnel: [w342] -> w338
          tunnel: w338 -> [w343]
          tunnel: w337 -> [w356]
          tunnel: [w355] -> w335
          tunnel: w336 -> [w354]
          frame #0 {
            n138 = local write "Connected?"(FALSE ("Connected?")) -> ()
          }
          frame #1 {
            w344 = 0
            n139 = Unbundle(w343) -> ("Switch to Safe State Ref"=w352:refnum<vi>, "Run Control Ref"=w351:refnum<vi>, "Stop Control Ref"=w350:refnum<vi>, "Update Control Configurations Ref"=w349:refnum<vi>, "Chatter Data Ref"=w348:refnum<vi>, "Max Acceleration Threshold Ref"=w347:refnum<vi>)
            n140 = property on="Controller Address" class="Str"("DisabledEnum"=w344) -> ()  [unwired: 2 in, 2 out]
            n141 = property on="Connect to Controller" class="Bool"("DisabledEnum"=w344) -> ()  [unwired: 2 in, 2 out]
            n142 = Build Array(w352, w351, w350, w349, w348, w347) -> (w346:refnum<vi>[])
            n143 = call "Set Enable State on Multiple Controls.vi"("Enable?"=FALSE, "Controls"=w346) -> ()  [unwired: 10 in]
          }
          frame #2 {
            n144 = Wait (ms)(milliseconds to wait=u32 1000) -> ()  [unwired: 1 out]
          }
          frame #3 {
            n145 = call "Enqueue Message.vi"("error in (no error)"=w356, "Message"="Connect", "Message Queue"=w354) -> ("error out"=w355:errorcluster)  [unwired: 7 in, 1 out]
          }
        }
        n146 = Merge Errors(w335) -> (w340:errorcluster)
      }
      frame Default {
        # "'Default' case only runs if there is a message that isn't defined in any of the other cases.  Output a programming error."
        n147 = Format Into String(format string="The invalid message string \"%s\" was received in the Message Handling Loop." ("Invalid Message Loop Message"), w362) -> (resulting string=w359:string)  [unwired: 2 in, 1 out]
        n148 = call <vilib>:"Error Cluster From Error Code.vi"("error message (\"\")"=w359, "error code (0)"=1) -> ("error out"=w360:errorcluster)  [unwired: 7 in]
      }
    }
    n149 = call <vilib>:"Clear Errors.vi"("error in (no error)"=w47) -> ("error out"=w46:errorcluster)  [unwired: 5 in, 1 out]
    n150 = call "UI Error Handler - Message Handler.vi"("error in (no error)"=w47, "Message Queue"=w48) -> ()  [unwired: 9 in, 1 out]
  }
  n151 = Tick Count (ms)() -> (millisecond timer value=w17:u32)
  n152 = while {
    tunnel: w29 -> [w364]
    tunnel: [w367] -> w39
    shift-right: [w365] -> w31
    shift-left: w37 -> [w366]
    stop <- w368 stop-if-true
    # "Event Handling Loop"
    n153 = event shown="[0] \"Connect to Controller\": Value Change" {
      selector: w366 -> [_ _ _ _ _ _ _ _]
      dyn-events: [_ _ _ _ _ _ _ _] -> w365
      timeout: _ -> [_ _ _ _ _ _ _ _]
      tunnel: [_ _ _ _ _ _ _ TRUE ("Discard?")] -> w369
      tunnel: w364 -> [w375 w378 w381 w384 w389 _ w394 _]
      tunnel: [w377 w380 w383 w386 w388 _ w397 _] -> w367
      tunnel: w364 -> [_ _ _ _ _ w393 _ _]
      event "Connect to Controller": Value Change {
        n154 = event-data() -> ()  [unwired: 1 in, 1 out]
        n155 = call "Enqueue Message.vi"("Message"="Connect", "Message Queue"=w375) -> ("error out"=w377:errorcluster)  [unwired: 8 in, 1 out]
      }
      event "Run Control": Value Change {
        n156 = event-data() -> ()  [unwired: 1 in, 1 out]
        n157 = call "Enqueue Message.vi"("Message"="Run Control", "Message Queue"=w378) -> ("error out"=w380:errorcluster)  [unwired: 8 in, 1 out]
      }
      event "Stop Control": Value Change {
        n158 = event-data() -> ()  [unwired: 1 in, 1 out]
        n159 = call "Enqueue Message.vi"("Message"="Stop Control", "Message Queue"=w381) -> ("error out"=w383:errorcluster)  [unwired: 8 in, 1 out]
      }
      event "Switch to Safe State": Value Change {
        n160 = event-data() -> ()  [unwired: 1 in, 1 out]
        n161 = call "Enqueue Message.vi"("Message"="Run Safe State", "Message Queue"=w384) -> ("error out"=w386:errorcluster)  [unwired: 8 in, 1 out]
      }
      event "Max Acceleration Threshold (g)": Value Change {
        n162 = event-data() -> ()  [unwired: 1 in, 1 out]
        n163 = call "Enqueue Message.vi"("Message Data"="Max Acceleration Threshold (g)", "Message"="Update Max Acceleration Threshold", "Message Queue"=w389) -> ("error out"=w388:errorcluster)  [unwired: 7 in, 1 out]
      }
      event "Tool Data File", "OK Button": Value Change {
        n164 = event-data() -> ()  [unwired: 1 in, 3 out]
        n165 = call "Enqueue Message.vi"("Message Data"="Tool Data File", "Message"="Update Tool Data", "Message Queue"=w393) -> ()  [unwired: 7 in, 2 out]
      }
      event "Exit": Value Change {
        w395 = TRUE  # Priority Message
        # "The UI Message Loop handles sending the Exit message to other loops."
        n166 = event-data() -> ()  [unwired: 1 in, 1 out]
        n167 = call "Enqueue Message.vi"("Priority Message? (F)"=w395, "Message"="Exit", "Message Queue"=w394) -> ("error out"=w397:errorcluster)  [unwired: 7 in, 1 out]
      }
      event User Event {
        # "The Message Handling Loop processed an \"Exit\" message, which fired this event to stop the Event Handling Loop."
        n168 = event-data() -> ()  [unwired: 1 in, 1 out]
      }
    }
    n169 = case shown="No Error" w367 {
      tunnel: [w370 TRUE ("Discard?")] -> w368
      tunnel: w369 -> [w370 _]
      tunnel: w364 -> [_ w371]
      frame No Error {
      }
      frame Error {
        # "On error, send Exit message, and stop loop."
        n170 = call "Enqueue Message.vi"("Priority Message? (F)"=TRUE ("Discard?"), "Message"="Exit", "Message Queue"=w371) -> ()  [unwired: 7 in, 2 out]
      }
    }
  }
  n171 = while {
    tunnel: w29 -> [w402]
    tunnel: "milliseconds to wait" -> [w407]
    shift-right: [w403] -> _
    shift-left: w21 -> [w404]
    tunnel: w18 -> [w406]
    tunnel: w22 -> [w405]
    shift-right: [w399] -> _
    shift-left: w17 -> [w401]
    stop <- w409 stop-if-true
    # "Only read monitoring variables if the UI Main VI is connected to the RT target"
    # "Only the 'Exit' message in the UI Message Loop can stop the Monitoring Loop."
    # "Monitoring Loop"
    n172 = Tick Count (ms)() -> (millisecond timer value=w399:u32)
    n173 = Subtract(x=w399, y=w401) -> (x-y=→"Loop execution":u32)
    n174 = local read "Connected?"() -> (w408:bool)
    n175 = case shown="True" w408 {
      tunnel: w402 -> [_ w524]
      tunnel: w407 -> [w411 w520]
      tunnel: w404 -> [_ w505]
      tunnel: w406 -> [_ w504]
      tunnel: w405 -> [_ w503]
      tunnel: [w410 w502] -> w403
      tunnel: w404 -> [w410 w502]
      tunnel: w402 -> [_ w501]
      frame False {
        n176 = Wait (ms)(milliseconds to wait=w411) -> ()  [unwired: 1 out]
      }
      frame True {
        (unwired) 1 ("length")
        (unwired) sgl 0.0 ("Tolerance")
        # "Serialize the shared variable calls to simplify the scheduling performed by LabVIEW at runtime"
        n177 = global read "Global - UI Stream and Variable Connections.vi" "Variable References"() -> (w522:T13)
        n178 = Unbundle By Name(w522) -> ("Current FPGA State"=w519:refnum<k21>, "Acceleration (grms)"=w516:refnum<k21>, "Acceleration Waveform"=w515:refnum<k21>, "Chatter"=w441:refnum<k21>, "tag acc"=w450:refnum<k21>, "tag video"=w449:refnum<k21>, "CPU Usage"=w415:refnum<k21>, "DMA FIFO Overflow?"=w414:refnum<k21>, "Free or Contiguous Memory"=w412:refnum<k21>)
        n179 = call "UI - Read Stream from RT.vi"("Message Queue"=w524) -> ("Message Received?"=w521:bool, "dup Message Queue"=w523:refnum<queue>)  [unwired: 8 in, 1 out]
        n180 = case shown="False" w521 {
          tunnel: w520 -> [w695 _]
          frame False {
            n181 = Wait Until Next ms Multiple(millisecond multiple=w695) -> ()  [unwired: 1 out]
          }
          frame True {
            # "If a message was received, immediately read again"
          }
        }
        n182 = shared-variable-read(w519) -> (w518:errorcluster, w508:T17)  [unwired: 1 in, 2 out]
        "Current FPGA State" <- w508
        n183 = shared-variable-read(w516, w518) -> (w517:errorcluster, w442:dbl[])  [unwired: 2 out]
        n184 = shared-variable-read(w515, w517) -> (w495:errorcluster, w432:waveform(dbl)[], w512:timestamp)  [unwired: 1 out]
        n185 = shared-variable-read(w441, w495) -> (w451:errorcluster, w494:bool[])  [unwired: 2 out]
        n186 = shared-variable-read(w450, w451) -> (w448:errorcluster, w439:string)  [unwired: 2 out]
        "tag acc" <- w439
        n187 = shared-variable-read(w449, w448) -> (w447:errorcluster, w435:string)  [unwired: 2 out]
        "tag spike" <- w435
        n188 = for {
          tunnel: w505 -> [w564] mode=indexing
          shift-right: [w566] -> w500
          shift-left: w447 -> [w565]
          tunnel: [w558] -> w478 mode=indexing
          tunnel: [w563] -> w492
          tunnel: w501 -> [w563]
          tunnel: w503 -> [w562]
          tunnel: w504 -> [w561]
          tunnel: [w559] -> w446
          tunnel: [w560] -> w437
          n189 = case "Message Cases" shown="\"Machine Data\"" w564 {
            tunnel: w565 -> [w573 w578 w585 w592 w600 w607 w614 w621 w628 w635 w642 w649 w656 w663 w670 w677 w682]
            tunnel: [w572 w577 w584 w590 w600 w607 w614 w621 w628 w635 w642 w649 w656 w663 w670 w677 w688] -> w566
            tunnel: [w567 w576 w581 w586 w595 w602 w609 w616 w623 w630 w638 w644 w652 w658 w665 w674 w678] -> w558
            tunnel: w562 -> [w569 w575 w583 w591 w596 w603 w610 w617 w624 w631 w636 w648 w650 w662 w666 w672 _]
            tunnel: w561 -> [_ _ _ _ _ _ _ _ _ _ _ _ _ _ _ _ w681]
            tunnel: [FALSE ("Triggger G1,G2, or G3") FALSE ("Triggger G1,G2, or G3") FALSE ("Triggger G1,G2, or G3") FALSE ("Triggger G1,G2, or G3") FALSE ("Triggger G1,G2, or G3") FALSE ("Triggger G1,G2, or G3") FALSE ("Triggger G1,G2, or G3") FALSE ("Triggger G1,G2, or G3") FALSE ("Triggger G1,G2, or G3") FALSE ("Triggger G1,G2, or G3") FALSE ("Triggger G1,G2, or G3") FALSE ("Triggger G1,G2, or G3") FALSE ("Triggger G1,G2, or G3") FALSE ("Triggger G1,G2, or G3") FALSE ("Triggger G1,G2, or G3") FALSE ("Triggger G1,G2, or G3") w687] -> w559
            tunnel: [_ _ _ _ _ _ _ _ _ _ _ _ _ _ _ _ w679] -> w560
            frame "Spindle Load" {
              # "maximum spindle power"
              # "Action 1 - Send an \"Update Display\" message indicating which button was pressed. Note that a string is sent as the Message Data along with the \"Update Display\" message."
              n190 = call "read_data_spindle_load_mt_connect (SubVI).vi"("error in (no error)"=w573, "URL"=w569) -> ("error out"=w572:errorcluster, "number"=w570:dbl[])  [unwired: 8 in]
              n191 = Multiply(x=1, y=w570) -> (x*y=w567:dbl[])
              "Spindle Load" <- w567
            }
            frame "Spindle Speed" {
              # "Action 2 - Send an \"Update Display\" message indicating which button was pressed. Note that a string is sent as the Message Data along with the \"Update Display\" message."
              n192 = call "read_data_speed_mt_connect (SubVI).vi"("error in (no error)"=w578, "URL"=w575) -> ("error out"=w577:errorcluster, "number"=w576:dbl[])  [unwired: 8 in]
            }
            frame "Feed Rate", Default {
              n193 = call "read_data_feed_mt_connect (SubVI).vi"("error in (no error)"=w585, "URL"=w583) -> ("error out"=w584:errorcluster, "appended array"=w581:dbl[])  [unwired: 8 in]
              n194 = Index Array(array=w581, index=0) -> (element=→"Feed":dbl)
            }
            frame "Position I" {
              n195 = call "read_data_linear_position_mt_connect (SubVI).vi"("error in (no error)"=w592, "URL"=w591) -> ("error out"=w590:errorcluster, "I, J,K,X, Y,Z"=w588:dbl[])  [unwired: 8 in]
              n196 = Index Array(array=w588, index=0) -> (element=w587:dbl)
              n197 = Build Array(w587) -> (w586:dbl[])
            }
            frame "Position J" {
              n198 = call "read_data_linear_position_mt_connect (SubVI).vi"("URL"=w596) -> ("I, J,K,X, Y,Z"=w598:dbl[])  [unwired: 9 in, 1 out]
              n199 = Index Array(array=w598, index=1) -> (element=w597:dbl)
              n200 = Build Array(w597) -> (w595:dbl[])
            }
            frame "Position K" {
              n201 = call "read_data_linear_position_mt_connect (SubVI).vi"("URL"=w603) -> ("I, J,K,X, Y,Z"=w605:dbl[])  [unwired: 9 in, 1 out]
              n202 = Index Array(array=w605, index=2) -> (element=w604:dbl)
              n203 = Build Array(w604) -> (w602:dbl[])
            }
            frame "Position X" {
              n204 = call "read_data_linear_position_mt_connect (SubVI).vi"("URL"=w610) -> ("I, J,K,X, Y,Z"=w612:dbl[])  [unwired: 9 in, 1 out]
              n205 = Index Array(array=w612, index=3) -> (element=w611:dbl)
              n206 = Build Array(w611) -> (w609:dbl[])
            }
            frame "Position Y" {
              n207 = call "read_data_linear_position_mt_connect (SubVI).vi"("URL"=w617) -> ("I, J,K,X, Y,Z"=w619:dbl[])  [unwired: 9 in, 1 out]
              n208 = Index Array(array=w619, index=4) -> (element=w618:dbl)
              n209 = Build Array(w618) -> (w616:dbl[])
            }
            frame "Position Z" {
              n210 = call "read_data_linear_position_mt_connect (SubVI).vi"("URL"=w624) -> ("I, J,K,X, Y,Z"=w626:dbl[])  [unwired: 9 in, 1 out]
              n211 = Index Array(array=w626, index=5) -> (element=w625:dbl)
              n212 = Build Array(w625) -> (w623:dbl[])
            }
            frame "Position A" {
              n213 = call "read_data_linear_angle_mt_connect (SubVI).vi"("URL"=w631) -> ("I, J,K,X, Y,Z"=w633:dbl[])  [unwired: 9 in, 1 out]
              n214 = Index Array(array=w633, index=0) -> (element=w632:dbl)
              n215 = Build Array(w632) -> (w630:dbl[])
            }
            frame "Position B" {
              n216 = call "read_data_linear_angle_mt_connect (SubVI).vi"("URL"=w636) -> ("I, J,K,X, Y,Z"=w640:dbl[])  [unwired: 9 in, 1 out]
              n217 = Index Array(array=w640, index=1) -> (element=w639:dbl)
              n218 = Build Array(w639) -> (w638:dbl[])
            }
            frame "Xload" {
              n219 = call "read_data_linear_loadX_mt_connect (SubVI).vi"("URL"=w648) -> ("I, J,K,X, Y,Z"=w646:dbl[])  [unwired: 9 in, 1 out]
              n220 = Index Array(array=w646, index=0) -> (element=w645:dbl)
              n221 = Build Array(w645) -> (w644:dbl[])
            }
            frame "Yload" {
              n222 = call "read_data_linear_loadX_mt_connect (SubVI).vi"("URL"=w650) -> ("I, J,K,X, Y,Z"=w654:dbl[])  [unwired: 9 in, 1 out]
              n223 = Index Array(array=w654, index=1) -> (element=w653:dbl)
              n224 = Build Array(w653) -> (w652:dbl[])
            }
            frame "Zload" {
              n225 = call "read_data_linear_loadX_mt_connect (SubVI).vi"("URL"=w662) -> ("I, J,K,X, Y,Z"=w659:dbl[])  [unwired: 9 in, 1 out]
              n226 = Index Array(array=w659, index=2) -> (element=w660:dbl)
              n227 = Build Array(w660) -> (w658:dbl[])
            }
            frame "Aload" {
              n228 = call "read_data_angle_loadmt_connect (SubVI).vi"("URL"=w666) -> ("I, J,K,X, Y,Z"=w668:dbl[])  [unwired: 9 in, 1 out]
              n229 = Index Array(array=w668, index=0) -> (element=w667:dbl)
              n230 = Build Array(w667) -> (w665:dbl[])
            }
            frame "Bload" {
              n231 = call "read_data_angle_loadmt_connect (SubVI).vi"("URL"=w672) -> ("I, J,K,X, Y,Z"=w671:dbl[])  [unwired: 9 in, 1 out]
              n232 = Index Array(array=w671, index=1) -> (element=w676:dbl)
              n233 = Build Array(w676) -> (w674:dbl[])
            }
            frame "Machine Data" {
              n234 = call "read_machine_parameters_mt_connect (SubVI).vi"("URL 2"=w681, "error in (no error) 3"=w682) -> ("error out 3"=w680:errorcluster, "Machine Data"=w679:T14)  [unwired: 7 in]
              n235 = Unbundle By Name(w679) -> ("Block of code being executed"=w689:string)
              "Block of code being executed" <- w689
              n236 = Unbundle By Name(w679) -> ("Tool_id"=→"Tool id":string, "Program Name"=w686:string)
              "Program Name" <- w686
              n237 = Decimal String To Number(string=w686) -> (number=w685:i32)  [unwired: 2 in, 1 out]
              n238 = call "check_G1_G2_G3.vi"("current line"=w689, "error in (no error)"=w680) -> ("Triggger G1,G2, or G3"=w687:bool, "error out (no error)"=w688:errorcluster)  [unwired: 7 in]
              n239 = To Double Precision Float(number=w685) -> (double precision float=w684:dbl)
              n240 = Build Array(w684) -> (w678:dbl[])
            }
          }
        }
        n241 = Or(x=w446, y="Save?") -> (x .or. y?=w445:bool)
        n242 = Boolean To (0,1)(Boolean=w494) -> (0, 1=w433:i16[])
        n243 = Equal?(x=w508, y=FPGA_state."Safe State") -> (x = y?=w510:bool)
        n244 = shared-variable-read(w412) -> (→"Free Physical Memory or Largest Contiguous Memory (bytes)":dbl)  [unwired: 1 in, 3 out]
        n245 = feedback #1(timestamp(0 s since 1904-01-01)) -> (w514:timestamp)
        n246 = feedback-in #1(w512) -> ()
        n247 = case shown="True" w510 {
          frame False {
            n248 = property on="Run Control" class="Bool"("DisabledEnum"=T7."Disabled and Grayed Out" ("Disabled")) -> ()  [unwired: 2 in, 2 out]
            n249 = property on="Stop Control" class="Bool"("DisabledEnum"=T7."Enabled" ("Disabled")) -> ()  [unwired: 2 in, 2 out]
          }
          frame True {
            n250 = property on="Run Control" class="Bool"("DisabledEnum"=T7."Enabled" ("Disabled")) -> ()  [unwired: 2 in, 2 out]
            n251 = property on="Stop Control" class="Bool"("DisabledEnum"=T7."Disabled and Grayed Out" ("Disabled")) -> ()  [unwired: 2 in, 2 out]
          }
        }
        n252 = Array Subset(array=w442, index=0, length=3) -> (w443:dbl[])
        n253 = Equal?(x=w512, y=w514) -> (x = y?=w444:bool)
        n254 = for {
          tunnel: w432 -> [w538] mode=indexing
          tunnel: [w536] -> w431 mode=indexing
          n255 = Unbundle By Name(w538) -> ("Y"=w537:dbl[])
          n256 = call "Analyze Acceleration (RT).vi"("Acceleration Waveform (SGL)"=w537) -> ("Acceleration (grms)"=w534:dbl)  [unwired: 8 in, 2 out]
          n257 = Format Into String(w534) -> (resulting string=w532:string)  [unwired: 3 in, 1 out]
          n258 = Equal?(x=w532, y="NaN") -> (x = y?=w530:bool)
          n259 = Equal?(x=w532, y="Inf") -> (x = y?=w531:bool)
          n260 = Or(x=w530, y=w531) -> (x .or. y?=w529:bool)
          n261 = case shown="False" w529 {
            tunnel: [w539 0] -> w536
            tunnel: w534 -> [w539 _]
            frame False {
            }
            frame True {
            }
          }
        }
        n262 = Array Size(array=w442) -> ()  [unwired: 1 out]
        n263 = Array To Cluster(array=w443) -> (cluster=→"ACC  (grms)":cluster{"[0]":dbl, "[1]":dbl, "[2]":dbl})
        n264 = control-ref of="STC Starrag"() -> (w471:refnum<vi>)
        n265 = case shown="False" w444 {
          tunnel: w432 -> [_ _]
          tunnel: w432 -> [w694 _]
          frame False {
            "Raw Waveform" <- w694
          }
          frame True {
          }
        }
        n266 = shared-variable-read(w414) -> (w422:errorcluster, →"DMA FIFO Overflow?":bool)  [unwired: 1 in, 2 out]
        n267 = shared-variable-read(w415, w422) -> (w421:T18)  [unwired: 3 out]
        n268 = for {
          tunnel: w421 -> [w526] mode=indexing
          tunnel: [w525] -> w420 mode=indexing
          n269 = Unbundle By Name(w526) -> ("Total (%)"=w525:dbl)
        }
        n270 = property on="Property Node" class="Bool (strict)"(reference=w471) -> ("Colors [4]"=w465:cluster{u32, u32}[])  [unwired: 1 in, 2 out]
        n271 = Array Size(array=w420) -> (size(s)=w419:i32)
        n272 = Bundle By Name(cluster=T16 {"Magnitude threshold"=0.0, "Tolerance"=0.0} ("Limits"), "Magnitude threshold"=sgl 0.00015, "Tolerance"=sgl 2.0) -> (w484:T16)
        n273 = Reshape Array(w420, 1 ("dimension size"), w419) -> (→"CPU Usage (%)":dbl[][])
        n274 = Index Array(array=w465, index=2) -> (element=w467:cluster{u32, u32})
        n275 = Bundle By Name(cluster=cluster{"G1 ":bool} {"G1 "=FALSE} ("G1 status"), "G1"=w445) -> (w452:cluster{"G1 ":bool})
        "output cluster" <- w452
        n276 = Array Subset(array=w442, index=3, length=3) -> (w454:dbl[])
        n277 = Build Array(w431) -> (w430:dbl[][])
        n278 = Transpose 2D Array(2D array=w430) -> (transposed array=w428:dbl[][])
        n279 = Index Array(array=w478, index (row)=1, index (col)=0 ("disabled index (col)")) -> (element=w479:dbl)
        "RPM" <- w479
        n280 = Bundle By Name(cluster=cluster{"rpm":sgl} {"rpm"=0.0} ("Cutting data"), "rpm"=w479) -> (w486:cluster{"rpm":sgl})
        n281 = Build Array(w442) -> (w497:dbl[][])
        n282 = Array To Cluster(array=w454) -> (cluster=→"Force (grms)":T4)
        n283 = Transpose 2D Array(2D array=w497) -> (transposed array=w496:dbl[][])
        n284 = Get Date/Time In Seconds() -> (seconds since 1Jan1904=w506:timestamp)
        n285 = Or(x="Save?", y=w446) -> (x .or. y?=w440:bool)
        n286 = Insert Into Array(array=w478, new element=w496) -> (w429:dbl[][])  [unwired: 2 in]
        n287 = Insert Into Array(array=w429, new element=w428) -> (w427:dbl[][])  [unwired: 2 in]
        n288 = case shown="False" w440 {
          tunnel: w439 -> [_ w545]
          tunnel: [w543 w548] -> w438
          tunnel: w437 -> [w544 w547]
          tunnel: w435 -> [_ w546]
          frame False {
            n289 = Bundle By Name(cluster=w544, "path_position"="Unavailable" ("Tool_id"), "Xload"="Unavailable" ("Tool_id")) -> (w543:T14)
          }
          frame True {
            n290 = Bundle By Name(cluster=w547, "path_position"=w545, "Xload"=w546) -> (w548:T14)
          }
        }
        n291 = Bundle("seconds since 1Jan1904"=w506, "appended array"=w427, "Machine Data"=w438) -> (w507:T19)  [unwired: 1 in]
        n292 = To Variant(anything=w507) -> (Variant=w498:variant)
        n293 = case shown="False" w440 {
          tunnel: ["Plot" ("Message") "Plot and Save" ("Message")] -> w499
          frame False {
          }
          frame True {
          }
        }
        n294 = Unbundle By Name(w437) -> ("Program status"=w426:string)
        n295 = case shown="\"READY\"" w426 {
          tunnel: [u32 16723242 u32 6618880 u32 16449369 u32 16449369 u32 16449369] -> w464
          frame "Stopped", Default {
          }
          frame "ACTIVE" {
          }
          frame "INTERRUPTED" {
          }
          frame "FEED_HOLD" {
          }
          frame "READY" {
          }
        }
        n296 = Bundle(cluster=w467, w464) -> (w468:cluster{u32, u32})  [unwired: 1 in]
        n297 = Insert Into Array(array=w465, index=0, new element #1=w468, new element #2=w468, new element #3=w468, new element #4=w468) -> (w466:cluster{u32, u32}[])
        n298 = property on="Property Node" class="Bool (strict)"(reference=w471, "Colors [4]"=w466) -> ()  [unwired: 1 in, 2 out]
        n299 = Equal?(x=w426, y="ACTIVE") -> (x = y?=w423:bool)
        n300 = case shown="True" w423 {
          tunnel: [sgl 0.0 ("Tolerance") sgl 1.0 ("Tolerance")] -> w424
          frame False {
          }
          frame True {
          }
        }
        n301 = Bundle By Name(cluster=cluster{"Number of teeth":sgl} {"Number of teeth"=0.0} ("Tool data"), "Number of teeth"=w424) -> (w488:cluster{"Number of teeth":sgl})
        n302 = Bundle By Name(cluster=T9 {"Tool data"={"Number of teeth"=2.0}, "Cutting data"={"rpm"=9898.0}, "Limits"={"Magnitude threshold"=0.0, "Tolerance"=1.0}, "G1 status"={"G1 "=FALSE}} ("Chatter Data"), "Tool data"=w488, "Cutting data"=w486, "Limits"=w484, "G1 status"=w452) -> (w480:T9)
        n303 = call "Enqueue Message.vi"("Message Data"=w480, "Message"="Update Control Configuration", "Message Queue"=w492) -> ()  [unwired: 7 in, 2 out]
        n304 = Index Array(array=w478, index (row)=0, index (col)=0 ("disabled index (col)")) -> (element=w475:dbl)
        n305 = call "Enqueue Message.vi"("error in (no error)"=w500, "Message Data"=w498, "Message"=w499, "Message Queue"=w492) -> ("error out"=w472:errorcluster)  [unwired: 6 in, 1 out]
        n306 = call "UI Error Handler - Monitoring.vi"("error in (no error)"=w472, "Message Queue"=w523) -> ()  [unwired: 9 in, 1 out]
        n307 = Greater?(x=w475, y="In-cut Power Threshold") -> (0:w460:bool)
        n308 = And(x=w460, y=w440) -> (x .and. y?=w459:bool)
        n309 = case shown="False" w459 {
          tunnel: w433 -> [_ w555]
          tunnel: [w554 w555] -> w463
          tunnel: i16[] [0, 0, 0] ("0, 1") -> [w554 _]
          frame False {
          }
          frame True {
          }
        }
        n310 = Not Equal To 0?(x=w463) -> (x != 0?=w462:bool[])
        n311 = Or Array Elements(Boolean array=w462) -> (logical OR=→"Chatter?":bool)
      }
    }
    n312 = global read "Global - All UI Loop Stop.vi" "All UI Loop Stop"() -> (w409:bool)
  }
  n313 = Unregister For Events(event registration refnum=w31, error in=w39) -> (error out=w32:errorcluster)
  n314 = Merge Errors(w32, w40) -> (w38:errorcluster)
  n315 = call "Destroy User Event - Stop.vi"("error in (no error)"=w38, "User Event - Stop"=w36) -> ("error out"=w30:errorcluster)  [unwired: 9 in]
  n316 = call <vilib>:"Simple Error Handler.vi"("error in (no error)"=w30) -> ()  [unwired: 4 in, 5 out]
